vi "GetDefaultTempConfig.vi"(2 "Error In":errorcluster, 3 "String":string) -> (0 "Error Out":errorcluster, 1 "TempConfig":T1)   [LabVIEW 2012]
uses:
  TempConfig.ctl
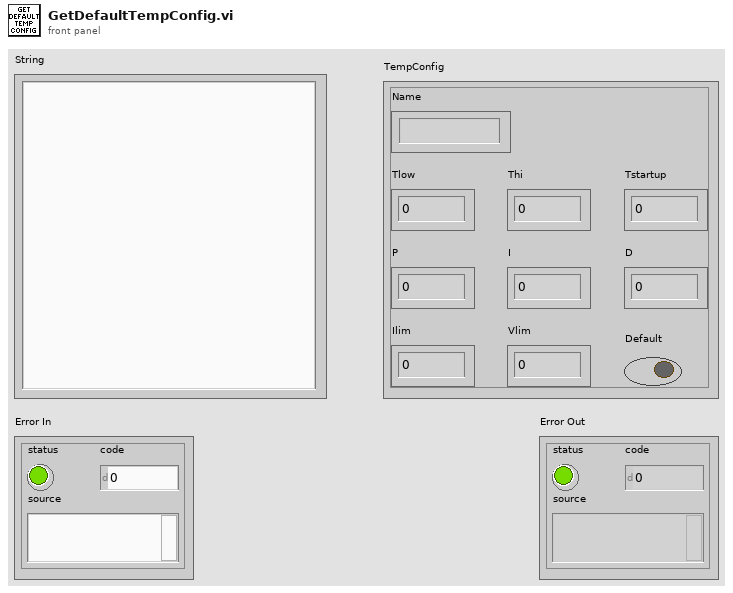
[diagram p1: front panel]
types:
  T1 = typedef "TempConfig.ctl" = cluster{"Name":string, "Thi":dbl, "Tlow":dbl, "Tstartup":dbl, "P":dbl, "I":dbl, "D":dbl, "Ilim":dbl, "Vlim":dbl, "Default":bool}
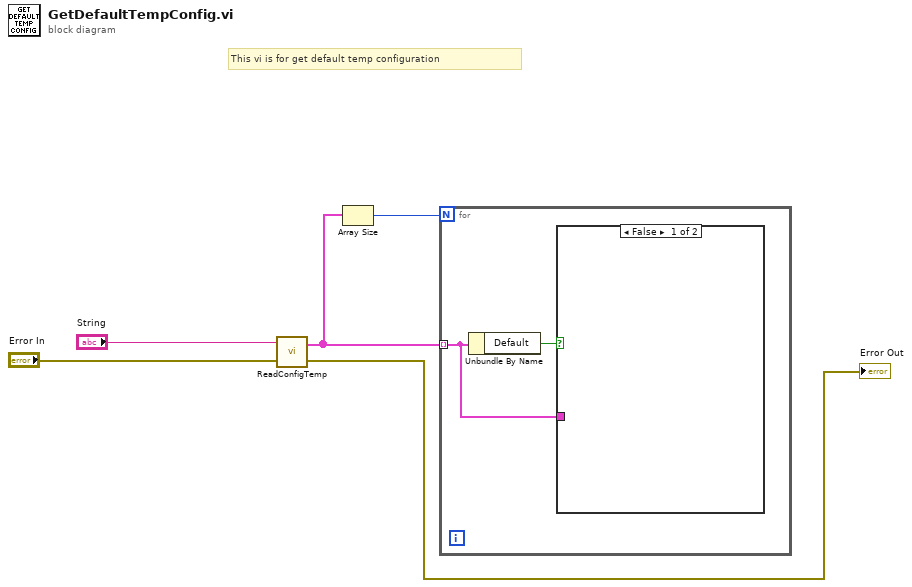
[diagram p0: block diagram]
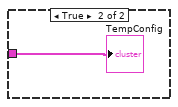
[diagram p2: hidden frame]
diagram:
  # "This vi is for get default temp configuration"
  n1 = call "ReadConfigTemp.vi"("Error In"="Error In", "Configs"="String") -> ("Error Out"=→"Error Out":errorcluster, "ConfigTemps"=w3:T1[])
  n2 = Array Size(array=w3) -> (size(s)=w2:i32)
  n3 = for {
    N: w2 -> [_]
    tunnel: w3 -> [w6] mode=indexing
    n4 = Unbundle By Name(w6) -> ("Default"=w7:bool)
    n5 = case shown="False" w7 {
      tunnel: w6 -> [_ w8]
      frame False {
      }
      frame True {
        "TempConfig" <- w8
      }
    }
  }
